vi "IR Sensor Init.vi"(8 "error in (no error)":errorcluster) -> (0 "error out":errorcluster, 3 "Ir Sensor":T1)   [LabVIEW 2020]
uses:
  <vilib>/High Genius/HG_WSI_Tookit/Dependencies/Library/Analog In/Analog In.lvclass
  C:/Program Files (x86)/National Instruments/LabVIEW 2020/vi.lib/High Genius/HG_WSI_Tookit/Dependencies/Library/HG_LIB/HG_LIB.lvclass
  <vilib>/High Genius/HG_WSI_Tookit/Dependencies/Library/HG_LIB/HG_LIB.lvclass
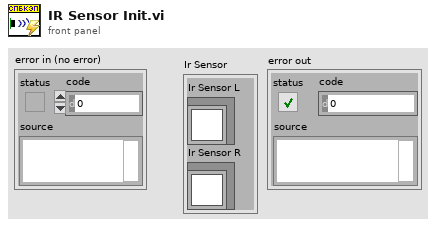
[diagram p1: front panel]
types:
  T1 = cluster{"Ir Sensor L":refnum<class "Analog In.lvclass">, "Ir Sensor R":refnum<class "Analog In.lvclass">}
  T2 = enum16{"DI", "DO", "AI", "Pulse", "PWM", "ISQ", "ENC", "CAN", "IIC", "IMU"}
  T3 = enum16{"0", "1", "2", "3", "4", "5", "6", "7", "8", "9", "10", "11", "12", "13", "14", "15", "16", "17", "18", "19", "20", "21", "22", "23", "24", "25"}
  T4 = cluster{"HG_LIB out":refnum<class "Analog In.lvclass">, "HG_LIB out":refnum<class "Analog In.lvclass">}
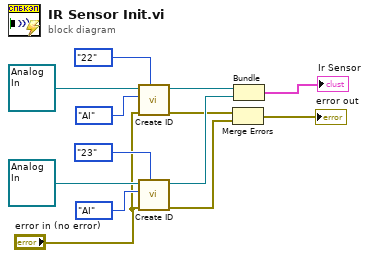
[diagram p0: block diagram]
diagram:
  n1 = call <vilib>:"Create ID.vi"("NO"=T3."22", "error in (no error)"="error in (no error)", "Function"=T2."AI", "HG_LIB in"=refnum<class "Analog In.lvclass"> refnum ("Analog In.lvclass")) -> ("error out"=w5:errorcluster, "HG_LIB out"=w8:refnum<class "Analog In.lvclass">)  [unwired: 6 in]
  n2 = call <vilib>:"Create ID.vi"("NO"=T3."23", "error in (no error)"="error in (no error)", "Function"=T2."AI", "HG_LIB in"=refnum<class "Analog In.lvclass"> refnum ("Analog In.lvclass")) -> ("error out"=w6:errorcluster, "HG_LIB out"=w7:refnum<class "Analog In.lvclass">)  [unwired: 6 in]
  n3 = Merge Errors(w5, w6) -> (→"error out":errorcluster)
  n4 = Bundle("HG_LIB out"=w8, "HG_LIB out"=w7) -> (→"Ir Sensor":T4)  [unwired: 1 in]
